vi "S2DS_CompileUserInfo.vi"(1 "User info":string[](array[string])) -> (0 "String":string)   [LabVIEW 2025]
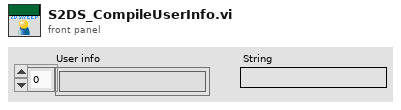
[diagram p1: front panel]
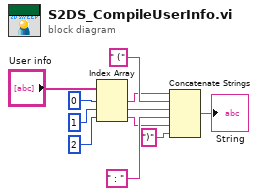
[diagram p0: block diagram]
diagram:
  n1 = Index Array(array="User info", index #1=0 ("index"), index #2=1 ("index"), index #3=2 ("index")) -> (element #1=w5:string, element #2=w6:string, element #3=w7:string)
  n2 = Concatenate Strings(w5, " (" ("string"), w6, " : " ("string"), w7, ")" ("string")) -> (→"String":string)
